vi "save_datapoint.vi"(0 "current value":dbl, 1 "Sample number":i32, 2 "current time of measurement":timestamp, 3 "Sensor type":T1) -> ()   [LabVIEW 2012]
uses:
  SensorTypes.ctl
  globalVariables.vi
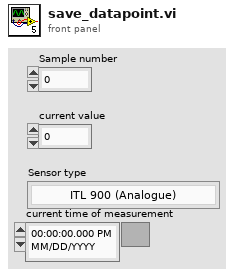
[diagram p1: front panel]
types:
  T1 = typedef "SensorTypes.ctl" = enum16{"ITL 900 (Analogue)", "CAB 300-C SP3 (CAN)", "xyz TODO (PWM)", "xyz TODO (LIN)", "xyz TODO (Analogue)"}
  T2 = typedef "TimeValue.ctl" = cluster{"Time of measurement":timestamp, "Current value":dbl}
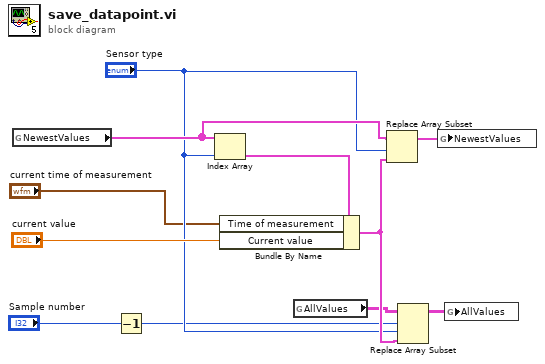
[diagram p0: block diagram]
diagram:
  n1 = global read "globalVariables.vi" "NewestValues"() -> (w6:T2[])
  n2 = Decrement(x="Sample number") -> (x-1=w1:i32)
  n3 = Index Array(array=w6, index="Sensor type") -> (element=w5:T2)
  n4 = Bundle By Name(cluster=w5, "Time of measurement"="current time of measurement", "Current value"="current value") -> (w9:T2)
  n5 = global read "globalVariables.vi" "AllValues"() -> (w8:T2[][])
  n6 = Replace Array Subset(array=w6, new element=w9, index="Sensor type") -> (w7:T2[])
  n7 = Replace Array Subset(array=w8, new element=w9, index (row)=w1, index (col)="Sensor type") -> (w10:T2[][])
  n8 = global write "globalVariables.vi" "NewestValues"(w7) -> ()
  n9 = global write "globalVariables.vi" "AllValues"(w10) -> ()
